vi "Read FPGA Target Name.vi"(8 "error in (no error)":errorcluster, 11 "Project in":refnum<class "Project.lvclass">) -> (0 "error out":errorcluster, 2 "FPGA Target Name":string="FPGA Target", 3 "Project out":refnum<class "Project.lvclass">)   [LabVIEW 2019, in "Project.lvclass"]
uses:
  Project.lvclass
  Project.lvclass/Project.ctl
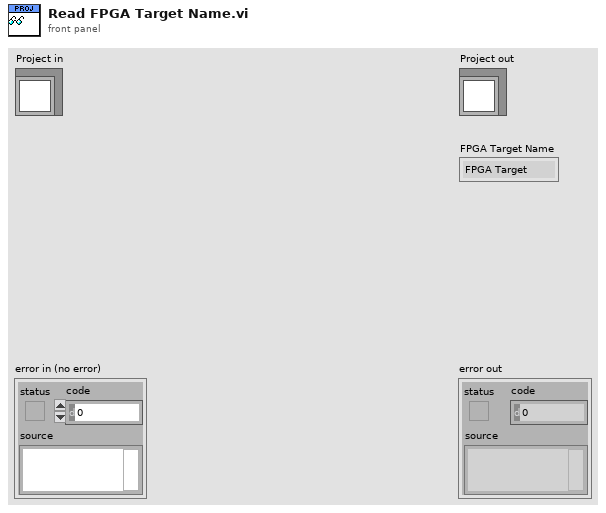
[diagram p1: front panel]
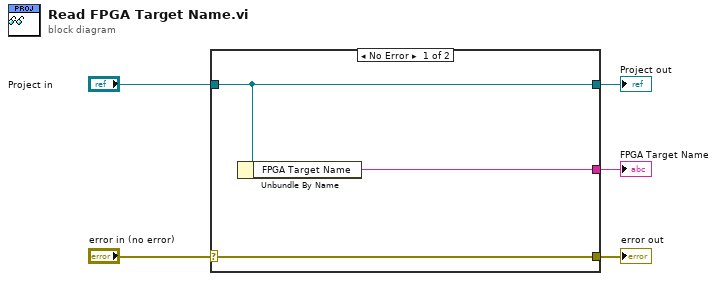
[diagram p0: block diagram]
diagram:
  n1 = case shown="No Error" "error in (no error)" {
    selector: "error in (no error)" -> [w8 w9]
    tunnel: [w8 w9] -> w4
    tunnel: [w7 w10] -> w2
    tunnel: "Project in" -> [w7 w10]
    tunnel: [w6 _] -> w1
    frame No Error {
      n2 = Unbundle By Name(w7) -> ("FPGA Target Name"=w6:string)
    }
    frame Error {
    }
  }
  "error out" <- w4
  "Project out" <- w2
  "FPGA Target Name" <- w1
